vi "Generate Digital Lines String(SAIN 1 PORT).vi"(9 "Port 2":dbl=2.0, 10 "Port":dbl=1.0, 11 "Device":dbl) -> (3 "lines":tag="Dev0/port1/line0,Dev0/port1/line1,Dev0/port1/line2,Dev0/port1/line3,Dev0/port1/line4,Dev0/port1/line5,Dev0/port1/line6,Dev0/port1/line7,Dev0/port2/line0,Dev0/port2/line1,Dev0/port2/line2,Dev0/port2/line3,Dev0/port2/line4,Dev0/port2/line5,Dev0/port2/line6,Dev0/port2/line7,")   [LabVIEW 2013]
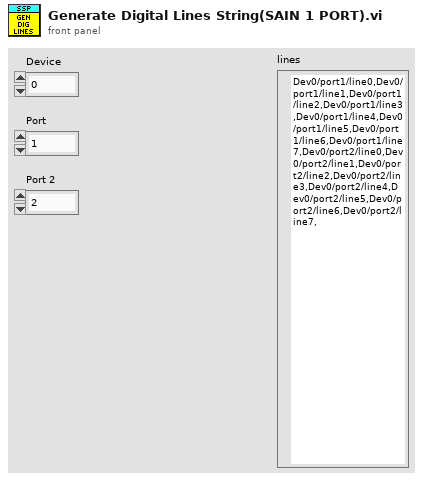
[diagram p1: front panel]
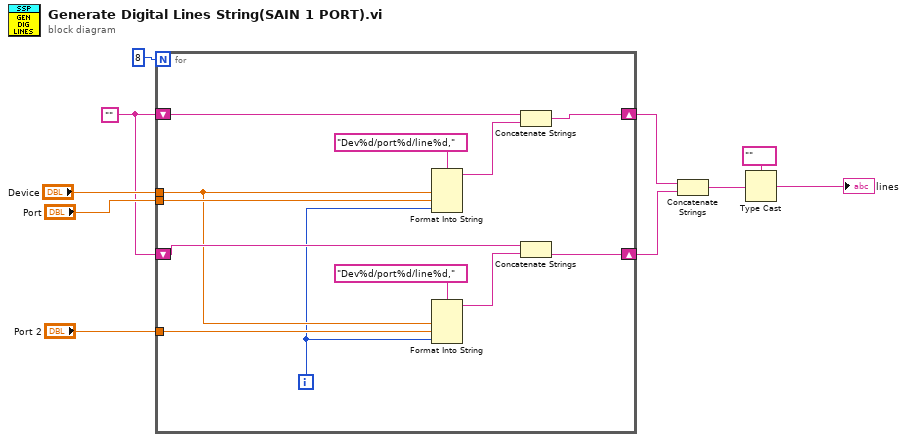
[diagram p0: block diagram]
diagram:
  w5 = ""
  n1 = for {
    N: 8 -> [_]
    shift-right: [w21] -> w3
    shift-left: w5 -> [w22]
    tunnel: "Device" -> [w13]
    tunnel: "Port" -> [w19]
    shift-right: [w15] -> w2
    shift-left: w5 -> [w14]
    tunnel: "Port 2" -> [w12]
    i -> [w11]
    n2 = Format Into String(format string="Dev%d/port%d/line%d,", w13, w19, w11) -> (resulting string=w18:string)  [unwired: 2 in, 1 out]
    n3 = Format Into String(format string="Dev%d/port%d/line%d,", w13, w12, w11) -> (resulting string=w17:string)  [unwired: 2 in, 1 out]
    n4 = Concatenate Strings(w22, w18) -> (w21:string)
    n5 = Concatenate Strings(w14, w17) -> (w15:string)
  }
  n6 = Concatenate Strings(w3, w2) -> (w1:string)
  n7 = Type Cast(type=tag "" ("*(type *) &x"), x=w1) -> (*(type *) &x=→"lines":tag)
